vi "ROI entry-Extract just ROI X and Y values.vi"(11 "Single ROI component data":dbl[](array[numeric])) -> (3 "X and Y values array":dbl[](array[numeric]))   [LabVIEW 2020]
panel:
  # "X1\nY1"
  # "X2\nY2"
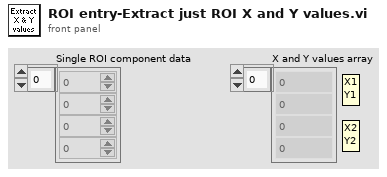
[diagram p1: front panel]
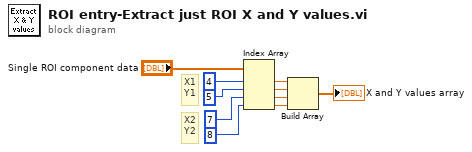
[diagram p0: block diagram]
diagram:
  # "X2\nY2"
  # "X1\nY1"
  n1 = Index Array(array="Single ROI component data", index #1=4 ("index"), index #2=5 ("index"), index #3=7 ("index"), index #4=8 ("index")) -> (element #1=w3:dbl, element #2=w4:dbl, element #3=w9:dbl, element #4=w10:dbl)
  n2 = Build Array(w3, w4, w9, w10) -> (→"X and Y values array":dbl[])
